vi "R30_1-FPGA.vi"() -> ()   [LabVIEW 2016]
uses:
  Glassman Control.ctl
  Faraday Cup Readback.ctl
  Aperture Readback.ctl
  Gate Valve Readback.ctl
  Glassman Readback.ctl
  <vilib>/LabVIEW Targets/FPGA/cRIO/shared/nicrio_ModuleControls/nicrio_cRIO-9871_BaudRateEnum.ctl
  <vilib>/LabVIEW Targets/FPGA/cRIO/shared/nicrio_ModuleControls/nicrio_cRIO-9871_ParityEnum.ctl
  <vilib>/LabVIEW Targets/FPGA/cRIO/shared/nicrio_ModuleControls/nicrio_cRIO-9871_StopBitsEnum.ctl
  <vilib>/LabVIEW Targets/FPGA/cRIO/shared/nicrio_ModuleControls/nicrio_cRIO-9871_DataBitsEnum.ctl
  <vilib>/Platform/TimedLoop/XDataNode/timing_clust.ctl
  <vilib>/Platform/TimedLoop/XDataNode/nitl_modes.ctl
  <vilib>/Platform/TimedLoop/XDataNode/wakeup.ctl
  <vilib>/rvi/FXPMathLib/basic elements/FxpIntAccumulator/subVIs/nifxpmath_IntAccumulator_SimConfig.ctl
  <vilib>/rvi/Emulation/niFpgaGetClockAttributes.vi
  <vilib>/rvi/Emulation/niFpgaSctlEmulationGetInTimedLoop.vi
  <vilib>/rvi/Emulation/niFpgaEmulationReportErrorSimple.vi
  <vilib>/rvi/eio/common/nirviEmuTemplateMethod_errors.vi
  <vilib>/rvi/Analysis/common/codeGenErrors/XNode/niFpgaXNodeCodeGenErrorHandle.vi
  <vilib>/rvi/Emulation/niFpgaCriticalErrorInLSC.vi
  <vilib>/rvi/FXPMathLib/basic elements/FxpIntAccumulator/simVIs/DllFxpIntAccumulator_sub.vi
  <vilib>/rvi/eio/common/nirviEmuTemplatePropertySet_errors.vi
  <vilib>/eio/EIONode/EIONode.xnode
  <vilib>/rvi/Analysis/measure/dc-rms/XNode/niFpgaDC-RMS.xnode
  <vilib>/Platform/TimedLoop/XDataNode/XDataNode.xnode
  <vilib>/rvi/FXPMathLib/basic elements/FxpIntAccumulator/XNode/nifxpmath_IntAccumulator.xnode
  <vilib>/rvi/FXPMathLib/FxpMul/XNode/nifxpmath_Multiplier.xnode
  <vilib>/eio/EIOPropertyNode/EIOPropertyNode.xnode
  <vilib>/eio/EIOMethodNode/EIOMethodNode.xnode
  <vilib>/Platform/TimedLoop/XDataNode/XDNodeRunTimeDep.lvlib
  <vilib>/rvi/FXPMathLib/sim/FxpSim.dll
  <vilib>/rvi/eio/common/nirviEmuTemplatePropertyGet_errors.vi
  <vilib>/rvi/eio/common/nirviEmuTemplatePropertyGet_noerrors.vi
  <vilib>/rvi/eio/common/nirviEmuTemplatePropertySet_noerrors.vi
panel:
  out "HV readback loop error":errorcluster
  out "Quad B I read":fxp<+/-,26,5>
  out "Quad A I read":fxp<+/-,26,5>
  out "ESA- Monitor":T1
  out "Mag Steerer Monitor":T1
  out "Y- Steerer Monitor":T1
  out "ESA+ Monitor":T1
  out "X+ Steerer Monitor":T1
  out "X- Steerer Monitor":T1
  out "Y+ Steerer Monitor":T1
  in  "RT error":bool
  out "GV Interlock loop error":errorcluster
  out "Vac cluster 3 Interlock":bool
  out "Vac cluster 2 Interlock":bool
  out "Vac cluster 1 Interlock":bool
  in  "Turbo 2 GV Actuator":bool
  in  "Beamline GV 2 Actuator":bool
  in  "Cryo Pump GV Actuator":bool
  in  "Beamline GV 1 Actuator":bool
  in  "Turbo 1 GV Actuator":bool
  in  "Switch Magnet GV Actuator":bool
  out "GV Status Loop error":errorcluster
  out "Cryo Pump GV Status":T2
  out "Turbo 2 GV Status":T2
  out "Beamline GV 2 Status":T2
  out "Turbo 1 GV Status":T2
  out "Beamline GV 1 Status":T2
  out "Switching Mag GV Status":T2
  in  "ESA- HV Enable":bool
  in  "ESA+ HV Enable":bool
  out "Switch Magnet Aperture Position":T3
  out "Detector Aperture Position":T3
  out "Detector FC Position":T4
  out "Switch Magnet FC Position":T4
  out "Actuator loop error":errorcluster
  in  "Y- Steerer V set":T5
  in  "Y+ Steerer V set":T5
  in  "X- Steerer V set":T5
  in  "X+ Steerer V set":T5
  in  "Quad B set":fxp<+/-,20,5>
  in  "Quad A set":fxp<+/-,20,5>
  in  "ESA Voltage set":fxp<+/-,20,5>
  out "HV control loop error":errorcluster
  out "Cryo Readback error":errorcluster
  out "Vacuum Gauge 1 error":errorcluster
  out "Vacuum Gauge 2 error":errorcluster
  out "Vacuum Gauge 3 error":errorcluster
  out "Switch Image Ion Gauge 1":u8[](array[numeric])
  out "Switch Image Convectron 1":u8[](array[numeric])
  out "Time since repurge":u8[](array[numeric])
  out "1st stage temp(k)":u8[](array[numeric])
  out "2nd stage":u8[](array[numeric])
  out "Time since pump on":u8[](array[numeric])
  out "Pump On":u8[](array[numeric])
  out "R30 ESA Convectron  1":u8[](array[numeric])
  out "R30 ESA Ion gauge 1":u8[](array[numeric])
  out "R30 Detector Convectron  1":u8[](array[numeric])
  out "R30 Detector Ion gauge 1":u8[](array[numeric])
  in  "Mag Steerer I-program":fxp<+/-,20,5> format="%.17g"
  in  "Switch magnet Aperture Actuator":bool
  in  "Detector Aperture Actuator":bool
  in  "Detector FC Actuator":bool
  in  "Switch magnet FC Actuator":bool
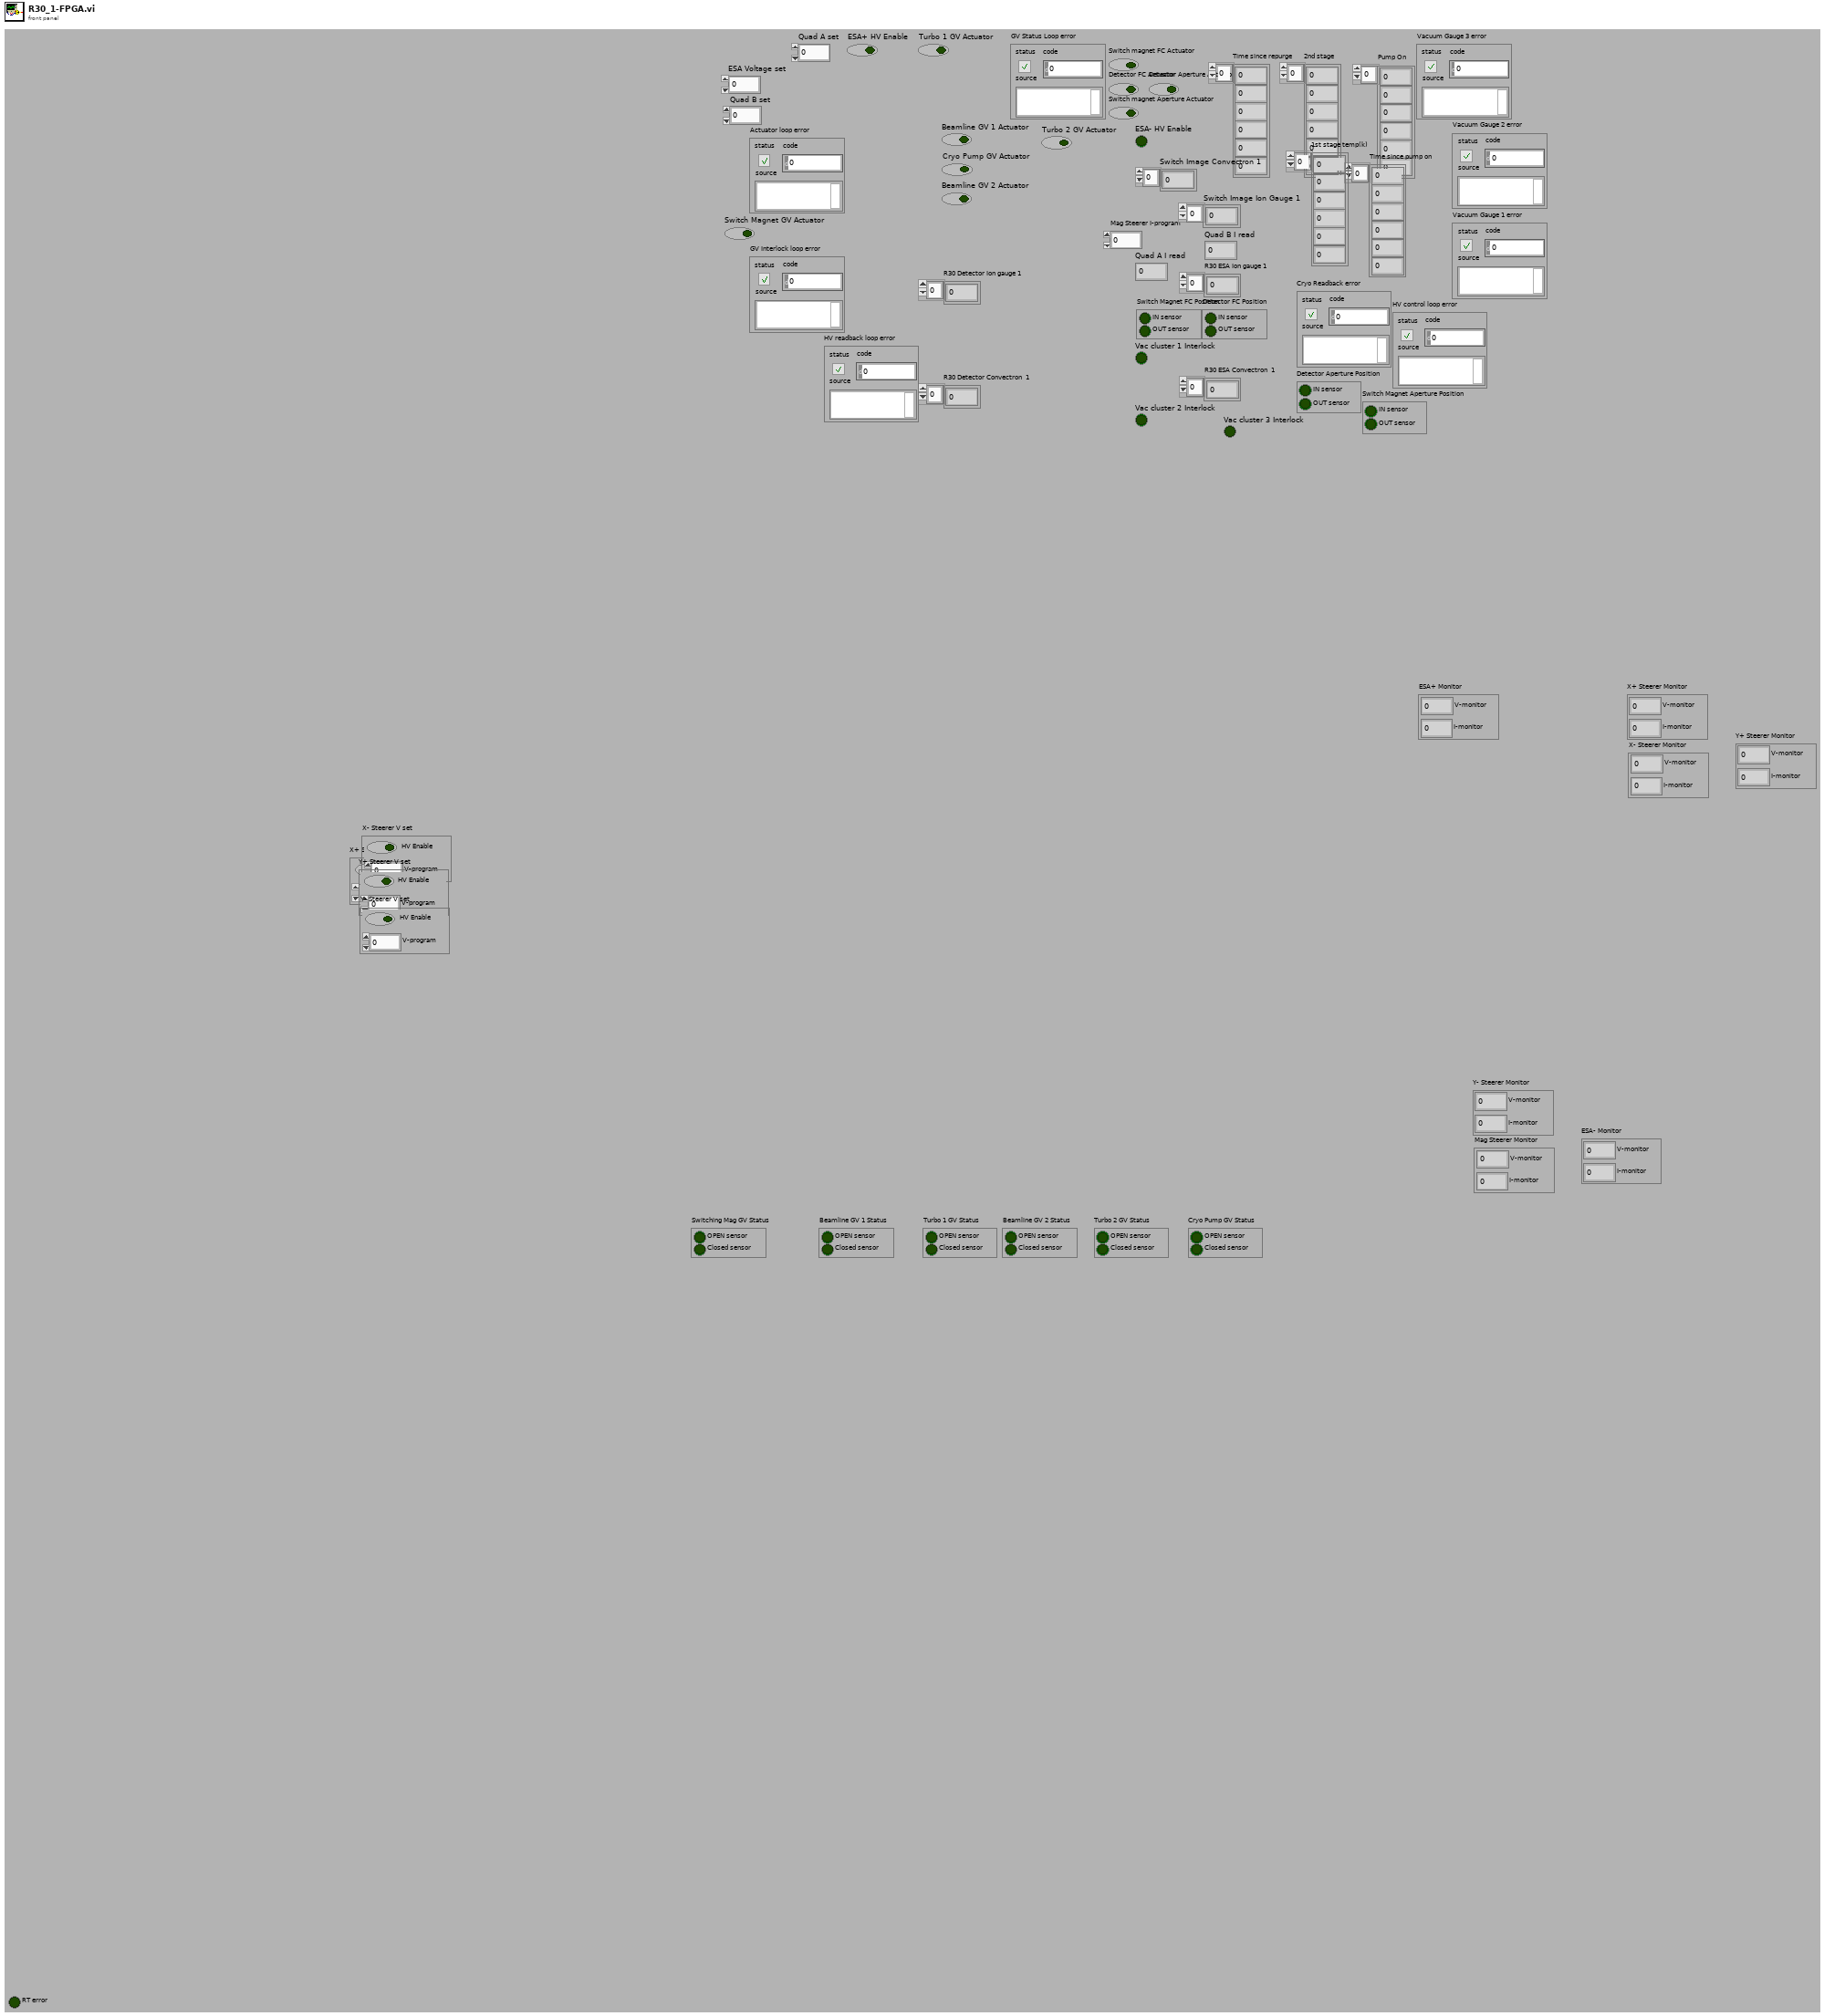
[diagram p1: front panel]
types:
  T1 = typedef "Glassman Readback.ctl" = cluster{"I-monitor":fxp<+/-,26,5>, "V-monitor":fxp<+/-,26,7>}
  T2 = typedef "Gate Valve Readback.ctl" = cluster{"OPEN sensor":bool, "Closed sensor":bool}
  T3 = typedef "Aperture Readback.ctl" = cluster{"IN sensor":bool, "OUT sensor":bool}
  T4 = typedef "Faraday Cup Readback.ctl" = cluster{"IN sensor":bool, "OUT sensor":bool}
  T5 = typedef "Glassman Control.ctl" = cluster{"V-program":fxp<+/-,20,7>, "HV Enable":bool}
  T6 = typedef "nicrio_cRIO-9871_StopBitsEnum.ctl" = enum8{"1", "1.5", "2"}
  T7 = typedef "nicrio_cRIO-9871_ParityEnum.ctl" = enum8{"None", "Odd", "Even", "Mark", "Space"}
  T8 = typedef "nicrio_cRIO-9871_DataBitsEnum.ctl" = enum8{"5", "6", "7", "8"}
  T9 = typedef "nicrio_cRIO-9871_BaudRateEnum.ctl" = enum16{"75 bps", "110 bps", "134 bps", "150 bps", "300 bps", "600 bps", "1200 bps", "1800 bps", "2400 bps", "4800 bps", "7200 bps", "9600 bps", "14.4 kbps", "19.2 kbps", "28.8 kbps", "38.4 kbps", "57.6 kbps", "115.2 kbps", "230.4 kbps", "460.8 kbps", "921.6 kbps"}
  T10 = typedef "XDNodeRunTimeDep.lvlib/timing_clust.ctl" = cluster{"Expected End [f-1]":u64, "Actual End [f-1]":u64, "Finished Late? [f-1]":bool, "Expected End [i-1]":u64, "Actual End [i-1]":u64, "Finished Late? [i-1]":bool, "Expected Start [i]":u64, "Actual Start [i]":u64, "Expected Start [f]":u64, "Actual Start [f]":u64, "Source Name":string, "Structure Name":string, "Period":i64, "Deadline":i64, "Offset":i64, "Start":i64, "Priority":i32, "Timeout":i32, "Mode":T11, "Wakeup Reason":T12, "Error":errorcluster, "Source Type":string, "Secondary Source Type":string, "Global End Time":u64, "Global Start Time":u64, "Frame Duration":u64, "Iteration Duration":u64, "Assigned CPU":i32, "I/O Scan Engine Mode":u32}
  T11 = typedef "XDNodeRunTimeDep.lvlib/nitl_modes.ctl" = enum32{"No Change", "Process missed periods, maintain original phase", "Discard missed periods, maintain original phase", "Process missed periods, ignore original phase", "Discard missed periods, ignore original phase"}
  T12 = typedef "XDNodeRunTimeDep.lvlib/wakeup.ctl" = enum32{"Normal", "Aborted", "Asynchronous wakeup", "Timing source error", "Timed loop error", "Timeout"}
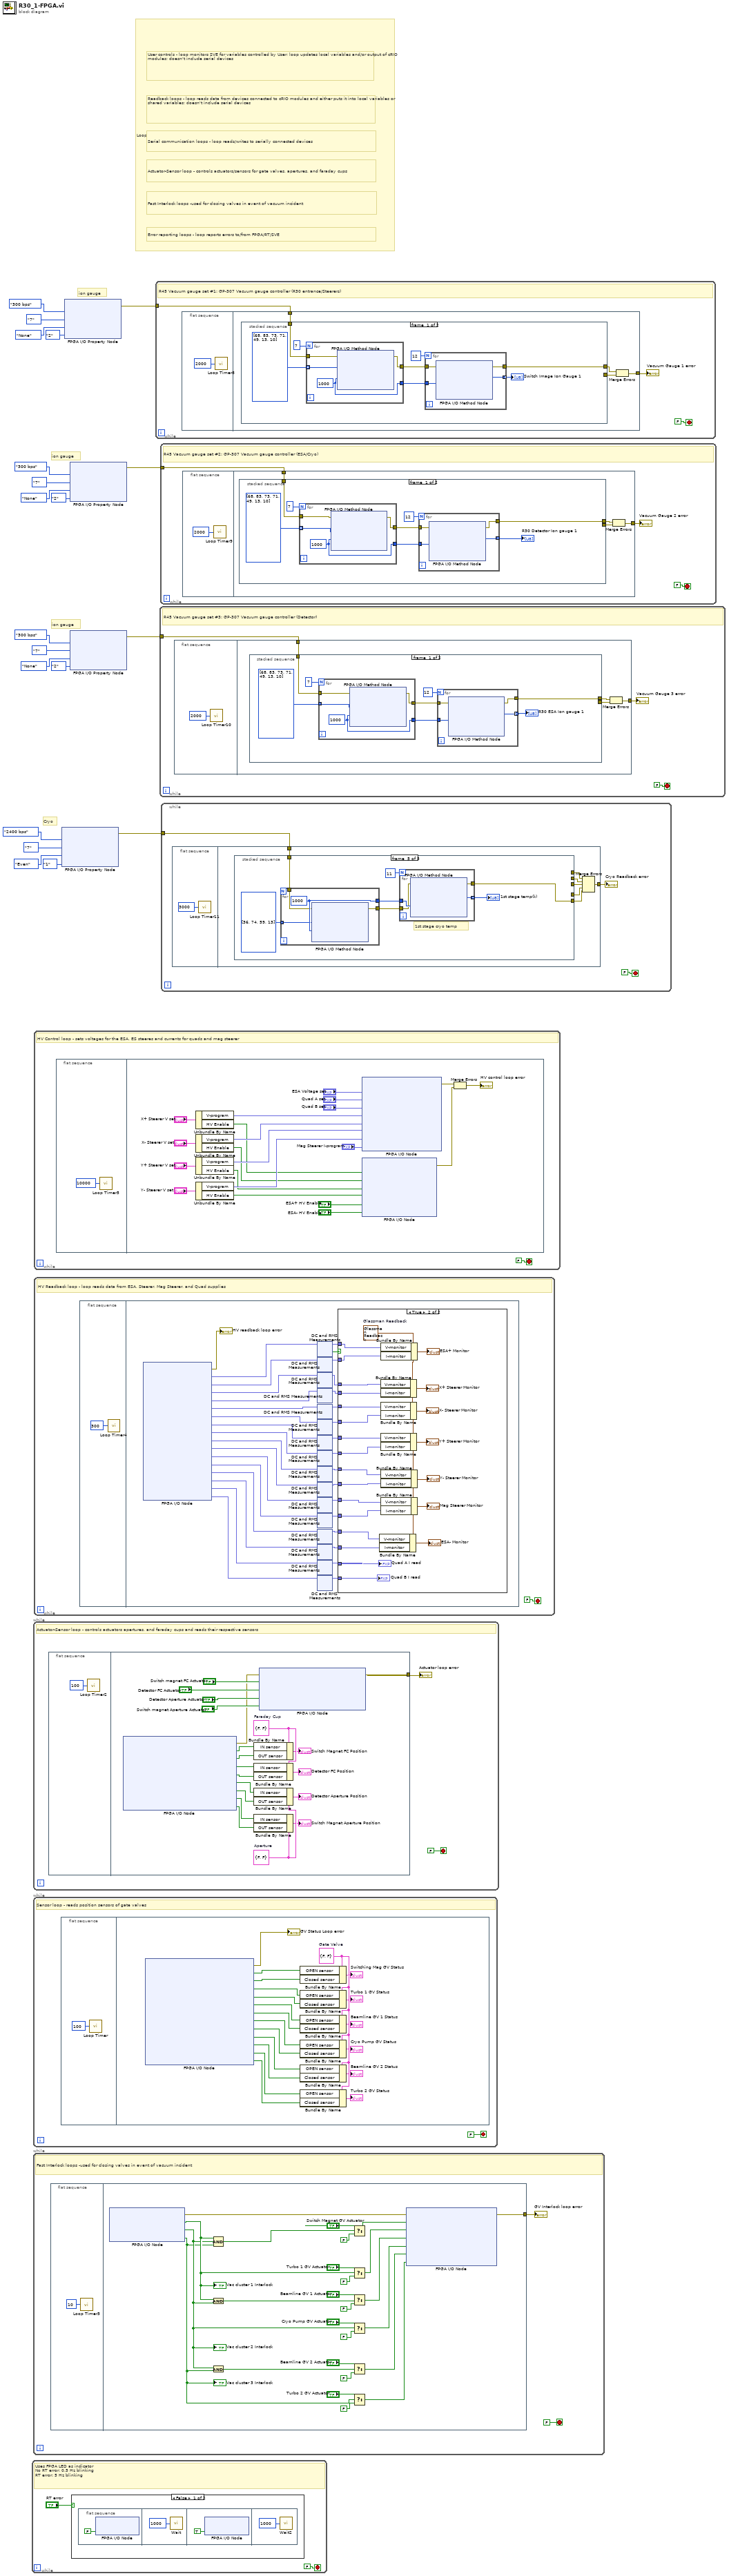
[diagram p0: block diagram]
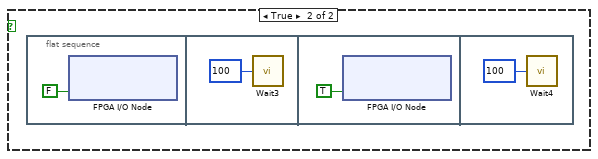
[diagram p2: hidden frame]
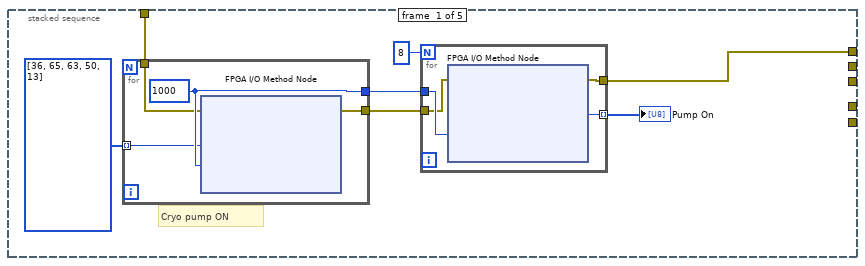
[diagram p3: hidden frame]
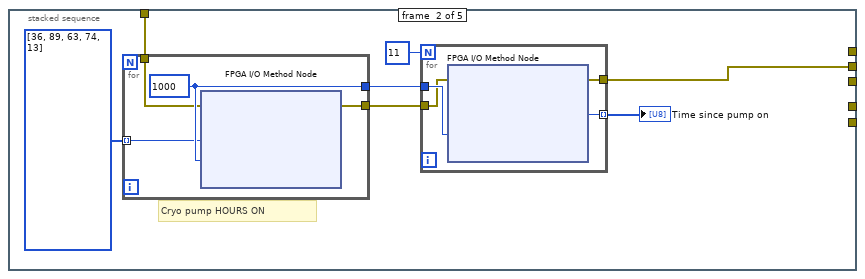
[diagram p4: hidden frame]
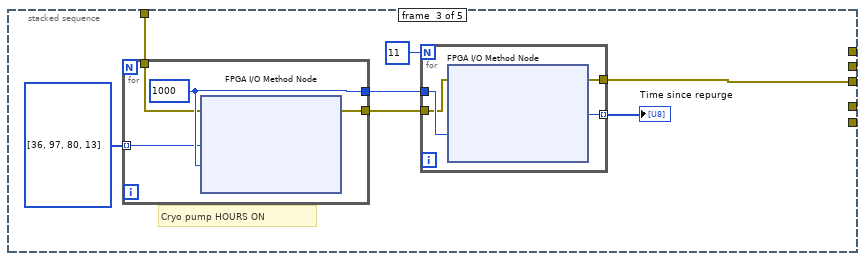
[diagram p5: hidden frame]
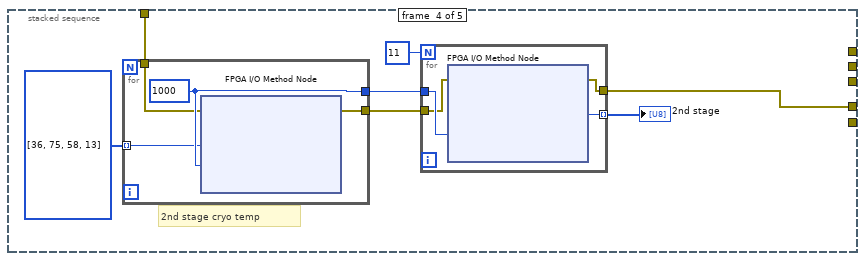
[diagram p6: hidden frame]
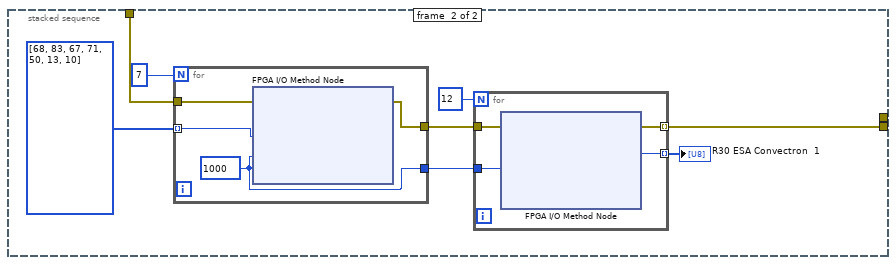
[diagram p7: hidden frame]
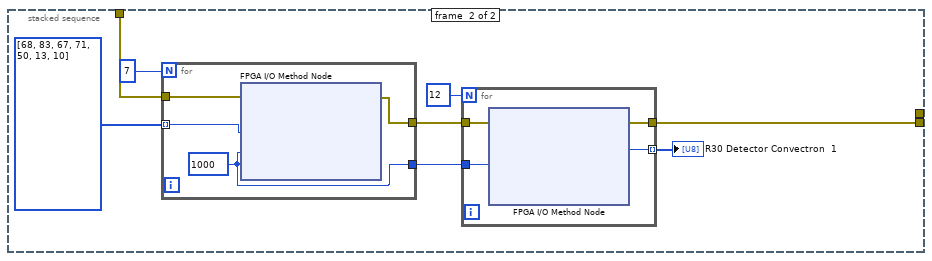
[diagram p8: hidden frame]
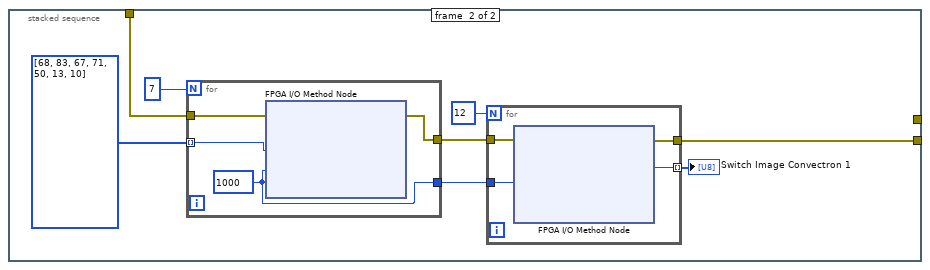
[diagram p9: hidden frame]
diagram:
  # "Actuator-Sensor loop - controls actuators/sensors for gate valves, apertures, and faraday cups"
  # "Fast Interlock loops -used for closing valves in event of vacuum incident"
  # "Error reporting loops - loop reports errors to/from FPGA/RT/SVE"
  # "Serial communication loops - loop reads/writes to serially connected devices"
  # "Readback loops - loop reads data from devices connected to cRIO modules and either puts it into local variables or shared variables; doesn't include serial devices"
  # "User controls - loop monitors SVE for variables controlled by User; loop updates local variables and/or output of cRIO modules; doesn't include serial devices"
  # "Loop legend - loops are color coded by responsibility"
  # "Cryo"
  # "ion gauge"
  # "ion gauge"
  # "ion gauge"
  n1 = while {
    stop <- FALSE stop-if-true
    # "Uses FPGA LED as indicator\nNo RT error: 0.5 Hz blinking\nRT error: 5 Hz blinking"
    n2 = case shown="False" "RT error" {
      frame False {
        n3 = flat-sequence {
          frame #0 {
            n4 = xnode "FPGA I/O Node"("FPGA LED"=FALSE) -> ()  [unwired: 1 in, 1 out]
          }
          frame #1 {
            n5 = call "Wait"("Count(mSec)"=u16 1000) -> ()  [unwired: 1 out]
          }
          frame #2 {
            n6 = xnode "FPGA I/O Node"("FPGA LED"=TRUE) -> ()  [unwired: 1 in, 1 out]
          }
          frame #3 {
            n7 = call "Wait2"("Count(mSec)"=u16 1000) -> ()  [unwired: 1 out]
          }
        }
      }
      frame True {
        n8 = flat-sequence {
          frame #0 {
            n9 = xnode "FPGA I/O Node"("FPGA LED"=FALSE) -> ()  [unwired: 1 in, 1 out]
          }
          frame #1 {
            n10 = call "Wait3"("Count(mSec)"=u16 100) -> ()  [unwired: 1 out]
          }
          frame #2 {
            n11 = xnode "FPGA I/O Node"("FPGA LED"=TRUE) -> ()  [unwired: 1 in, 1 out]
          }
          frame #3 {
            n12 = call "Wait4"("Count(mSec)"=u16 100) -> ()  [unwired: 1 out]
          }
        }
      }
    }
  }
  n13 = while {
    stop <- FALSE stop-if-true
    # "Fast Interlock loops -used for closing valves in event of vacuum incident"
    n14 = flat-sequence {
      tunnel: [w34] -> w31
      frame #0 {
        n15 = call "Loop Timer3"("Count(uSec)"=u32 10) -> ()  [unwired: 1 out]
      }
      frame #1 {
        n16 = xnode "FPGA I/O Node"() -> ("error out"=w59:errorcluster, "Vac cluster 1 Interlock"=w41:bool, "Vac cluster 2 Interlock"=w40:bool, "Vac cluster 3 Interlock"=w39:bool)  [unwired: 4 in, 3 out]
        "Vac cluster 1 Interlock" <- w41
        "Vac cluster 2 Interlock" <- w40
        "Vac cluster 3 Interlock" <- w39
        n17 = And(x=w41, y=w40) -> (x .and. y?=w45:bool)
        n18 = And(x=w40, y=w39) -> (x .and. y?=w52:bool)
        n19 = Compound Arithmetic op=AND(w41, w40, w39) -> (w36:bool)
        n20 = Select(t="Switch Magnet GV Actuator", s=w36, f=FALSE) -> (s? t:f=w35:bool)
        n21 = Select(t="Turbo 1 GV Actuator", s=w41, f=FALSE) -> (s? t:f=w43:bool)
        n22 = Select(t="Beamline GV 1 Actuator", s=w45, f=FALSE) -> (s? t:f=w47:bool)
        n23 = Select(t="Cryo Pump GV Actuator", s=w40, f=FALSE) -> (s? t:f=w50:bool)
        n24 = Select(t="Beamline GV 2 Actuator", s=w52, f=FALSE) -> (s? t:f=w54:bool)
        n25 = Select(t="Turbo 2 GV Actuator", s=w39, f=FALSE) -> (s? t:f=w57:bool)
        n26 = xnode "FPGA I/O Node"("error in"=w59, "Switch Magnet GV Actuator"=w35, "Turbo 1 GV Actuator"=w43, "Beamline GV 1 Actuator"=w47, "Cryo Pump GV Actuator"=w50, "Beamline GV 2 Actuator"=w54, "Turbo 2 GV Actuator"=w57) -> ("error out"=w34:errorcluster)  [unwired: 6 in, 6 out]
      }
    }
    "GV Interlock loop error" <- w31
  }
  n27 = while {
    stop <- FALSE stop-if-true
    # "Actuator-Sensor loop - controls actuators apertures, and faraday cups and reads their respective sensors"
    n28 = flat-sequence {
      tunnel: [w80] -> w60
      frame #0 {
        n29 = call "Loop Timer2"("Count(mSec)"=u32 100 ("Count(uSec)")) -> ()  [unwired: 1 out]
      }
      frame #1 {
        w69 = T3 {"IN sensor"=FALSE, "OUT sensor"=FALSE}  # Aperture
        w72 = T4 {"IN sensor"=FALSE, "OUT sensor"=FALSE}  # Faraday Cup
        n30 = xnode "FPGA I/O Node"() -> ("error out"=w77:errorcluster, "Switch Magnet FC IN sensor"=w76:bool, "Switch Magnet FC OUT sensor"=w75:bool, "Detector FC IN sensor"=w74:bool, "Detector FC OUT sensor"=w73:bool, "Detector Aperture IN sensor"=w65:bool, "Detector Aperture OUT sensor"=w66:bool, "Switch Magnet Aperture IN sensor"=w67:bool, "Switch Magnet Aperture OUT sensor"=w68:bool)  [unwired: 9 in, 8 out]
        n31 = Bundle By Name(cluster=w72, "IN sensor"=w76, "OUT sensor"=w75) -> (→"Switch Magnet FC Position":T4)
        n32 = Bundle By Name(cluster=w72, "IN sensor"=w74, "OUT sensor"=w73) -> (→"Detector FC Position":T4)
        n33 = Bundle By Name(cluster=w69, "IN sensor"=w65, "OUT sensor"=w66) -> (→"Detector Aperture Position":T3)
        n34 = Bundle By Name(cluster=w69, "IN sensor"=w67, "OUT sensor"=w68) -> (→"Switch Magnet Aperture Position":T3)
        n35 = xnode "FPGA I/O Node"("error in"=w77, "Switch Magnet FC Actuator"="Switch magnet FC Actuator", "Detector FC Actuator"="Detector FC Actuator", "Detector Aperture Acutator"="Detector Aperture Actuator", "Switch Magnet Aperture Actuator"="Switch magnet Aperture Actuator") -> ("error out"=w80:errorcluster)  [unwired: 4 in, 4 out]
      }
    }
    "Actuator loop error" <- w60
  }
  n36 = while {
    stop <- FALSE stop-if-true
    # "Sensor loop - reads position sensors of gate valves"
    n37 = flat-sequence {
      frame #0 {
        n38 = call "Loop Timer"("Count(mSec)"=u32 100 ("Count(uSec)")) -> ()  [unwired: 1 out]
      }
      frame #1 {
        w103 = T2 {"OPEN sensor"=FALSE, "Closed sensor"=FALSE}  # Gate Valve
        n39 = xnode "FPGA I/O Node"() -> ("error out"=→"GV Status Loop error":errorcluster, "Swtich Magnet GV OPEN Sensor"=w102:bool, "Swtich Magnet GV CLOSED Sensor"=w101:bool, "Turbo 1 GV OPEN sensor"=w100:bool, "Turbo 1 GV CLOSED sensor"=w99:bool, "Beamline GV 1 OPEN sensor"=w98:bool, "Beamline GV 1 CLOSED sensor"=w97:bool, "Cryo Pump GV OPEN sensor"=w96:bool, "Cryo Pump GV CLOSED sensor"=w95:bool, "Beamline GV 2 OPEN sensor"=w94:bool, "Beamline GV 2 CLOSED sensor"=w93:bool, "Turbo 2 GV OPEN sensor"=w92:bool, "Turbo 2 GV CLOSED sensor"=w91:bool)  [unwired: 13 in, 12 out]
        n40 = Bundle By Name(cluster=w103, "OPEN sensor"=w102, "Closed sensor"=w101) -> (→"Switching Mag GV Status":T2)
        n41 = Bundle By Name(cluster=w103, "OPEN sensor"=w100, "Closed sensor"=w99) -> (→"Turbo 1 GV Status":T2)
        n42 = Bundle By Name(cluster=w103, "OPEN sensor"=w98, "Closed sensor"=w97) -> (→"Beamline GV 1 Status":T2)
        n43 = Bundle By Name(cluster=w103, "OPEN sensor"=w96, "Closed sensor"=w95) -> (→"Cryo Pump GV Status":T2)
        n44 = Bundle By Name(cluster=w103, "OPEN sensor"=w94, "Closed sensor"=w93) -> (→"Beamline GV 2 Status":T2)
        n45 = Bundle By Name(cluster=w103, "OPEN sensor"=w92, "Closed sensor"=w91) -> (→"Turbo 2 GV Status":T2)
      }
    }
  }
  n46 = while {
    stop <- FALSE stop-if-true
    # "HV Control loop - sets voltages for the ESA, ES steeres and currents for quads and mag steerer"
    n47 = flat-sequence {
      frame #0 {
        n48 = call "Loop Timer5"("Count(Ticks)"=u32 10000 ("Count(mSec)")) -> ()  [unwired: 1 out]
      }
      frame #1 {
        n49 = Unbundle By Name("X+ Steerer V set") -> ("V-program"=w118:fxp<+/-,20,7>, "HV Enable"=w111:bool)
        n50 = Unbundle By Name("X- Steerer V set") -> ("V-program"=w117:fxp<+/-,20,7>, "HV Enable"=w112:bool)
        n51 = Unbundle By Name("Y+ Steerer V set") -> ("V-program"=w116:fxp<+/-,20,7>, "HV Enable"=w113:bool)
        n52 = Unbundle By Name("Y- Steerer V set") -> ("V-program"=w115:fxp<+/-,20,7>, "HV Enable"=w114:bool)
        n53 = xnode "FPGA I/O Node"("X+ Steerer HV Enable"=w111, "X- Steerer HV Enable"=w112, "Y+ Steerer HV Enable"=w113, "Y- Steerer HV Enable"=w114, "ESA+ HV Enable"="ESA+ HV Enable", "ESA- HV Enable"="ESA- HV Enable") -> ("error out"=w109:errorcluster)  [unwired: 7 in, 6 out]
        n54 = xnode "FPGA I/O Node"("ESA Voltage set"="ESA Voltage set", "Quad A set"="Quad A set", "Quad B set"="Quad B set", "X+ Steerer V set"=w118, "X- Steerer V set"=w117, "Y+ Steerer V set"=w116, "Y- Steerer V set"=w115, "Mag Steerer I-program"="Mag Steerer I-program") -> ("error out"=w126:errorcluster)  [unwired: 9 in, 8 out]
        n55 = Merge Errors(w126, w109) -> (→"HV control loop error":errorcluster)
      }
    }
  }
  n56 = while {
    stop <- FALSE stop-if-true
    # "HV Readback loop - loop reads data from ESA, Steerer, Mag Steerer, and Quad supplies"
    n57 = flat-sequence {
      frame #0 {
        n58 = call "Loop Timer4"("Count(Ticks)"=u32 300) -> ()  [unwired: 1 out]
      }
      frame #1 {
        n59 = xnode "FPGA I/O Node"() -> ("error out"=→"HV readback loop error":errorcluster, "ESA+ V read"=w154:fxp<+/-,26,5>, "ESA+ I read"=w153:fxp<+/-,26,5>, "X+ Steerer V read"=w152:fxp<+/-,26,5>, "X+ Steerer I read"=w151:fxp<+/-,26,5>, "X- Steerer V read"=w150:fxp<+/-,26,5>, "X- Steerer I read"=w149:fxp<+/-,26,5>, "Y+ Steerer V read"=w148:fxp<+/-,26,5>, "Y+ Steerer I read"=w147:fxp<+/-,26,5>, "Y- Steerer V read"=w140:fxp<+/-,26,5>, "Y- Steerer I read"=w139:fxp<+/-,26,5>, "Mag Steerer V read"=w138:fxp<+/-,26,5>, "Mag Steerer I read"=w137:fxp<+/-,26,5>, "ESA- V read"=w136:fxp<+/-,26,5>, "ESA- I read"=w135:fxp<+/-,26,5>, "Quad A I read"=w134:fxp<+/-,26,5>, "Quad B I read"=w133:fxp<+/-,26,5>)  [unwired: 17 in, 16 out]
        n60 = xnode "DC and RMS Measurements"("input data"=w154) -> ("DC"=w162:fxp<+/-,26,5>, "output valid"=w163:bool)  [unwired: 1 in]
        n61 = xnode "DC and RMS Measurements"("input data"=w153) -> ("DC"=w161:fxp<+/-,26,5>)  [unwired: 1 in, 1 out]
        n62 = xnode "DC and RMS Measurements"("input data"=w152) -> ("DC"=w160:fxp<+/-,26,5>)  [unwired: 1 in, 1 out]
        n63 = xnode "DC and RMS Measurements"("input data"=w151) -> ("DC"=w159:fxp<+/-,26,5>)  [unwired: 1 in, 1 out]
        n64 = xnode "DC and RMS Measurements"("input data"=w150) -> ("DC"=w158:fxp<+/-,26,5>)  [unwired: 1 in, 1 out]
        n65 = xnode "DC and RMS Measurements"("input data"=w149) -> ("DC"=w157:fxp<+/-,26,5>)  [unwired: 1 in, 1 out]
        n66 = xnode "DC and RMS Measurements"("input data"=w148) -> ("DC"=w156:fxp<+/-,26,5>)  [unwired: 1 in, 1 out]
        n67 = xnode "DC and RMS Measurements"("input data"=w147) -> ("DC"=w155:fxp<+/-,26,5>)  [unwired: 1 in, 1 out]
        n68 = xnode "DC and RMS Measurements"("input data"=w140) -> ("DC"=w146:fxp<+/-,26,5>)  [unwired: 1 in, 1 out]
        n69 = xnode "DC and RMS Measurements"("input data"=w139) -> ("DC"=w145:fxp<+/-,26,5>)  [unwired: 1 in, 1 out]
        n70 = xnode "DC and RMS Measurements"("input data"=w138) -> ("DC"=w144:fxp<+/-,26,5>)  [unwired: 1 in, 1 out]
        n71 = xnode "DC and RMS Measurements"("input data"=w137) -> ("DC"=w143:fxp<+/-,26,5>)  [unwired: 1 in, 1 out]
        n72 = xnode "DC and RMS Measurements"("input data"=w136) -> ("DC"=w142:fxp<+/-,26,5>)  [unwired: 1 in, 1 out]
        n73 = xnode "DC and RMS Measurements"("input data"=w135) -> ("DC"=w141:fxp<+/-,26,5>)  [unwired: 1 in, 1 out]
        n74 = xnode "DC and RMS Measurements"("input data"=w134) -> ("DC"=w132:fxp<+/-,26,5>)  [unwired: 1 in, 1 out]
        n75 = xnode "DC and RMS Measurements"("input data"=w133) -> ("DC"=w131:fxp<+/-,26,5>)  [unwired: 1 in, 1 out]
        n76 = case shown="True" w163 {
          tunnel: w162 -> [_ w987]
          tunnel: w161 -> [_ w986]
          tunnel: w160 -> [_ w982]
          tunnel: w159 -> [_ w981]
          tunnel: w158 -> [_ w980]
          tunnel: w157 -> [_ w979]
          tunnel: w156 -> [_ w977]
          tunnel: w155 -> [_ w976]
          tunnel: w146 -> [_ w972]
          tunnel: w145 -> [_ w971]
          tunnel: w144 -> [_ w970]
          tunnel: w143 -> [_ w969]
          tunnel: w142 -> [_ w968]
          tunnel: w141 -> [_ w967]
          tunnel: w132 -> [_ w965]
          tunnel: w131 -> [_ w964]
          frame False {
          }
          frame True {
            w966 = T1 {"I-monitor"=0.0, "V-monitor"=0.0}  # Glassman Readback
            n77 = Bundle By Name(cluster=w966, "V-monitor"=w968, "I-monitor"=w967) -> (→"ESA- Monitor":T1)
            n78 = Bundle By Name(cluster=w966, "V-monitor"=w982, "I-monitor"=w981) -> (→"X+ Steerer Monitor":T1)
            n79 = Bundle By Name(cluster=w966, "V-monitor"=w980, "I-monitor"=w979) -> (→"X- Steerer Monitor":T1)
            n80 = Bundle By Name(cluster=w966, "V-monitor"=w977, "I-monitor"=w976) -> (→"Y+ Steerer Monitor":T1)
            n81 = Bundle By Name(cluster=w966, "V-monitor"=w987, "I-monitor"=w986) -> (→"ESA+ Monitor":T1)
            n82 = Bundle By Name(cluster=w966, "V-monitor"=w972, "I-monitor"=w971) -> (→"Y- Steerer Monitor":T1)
            n83 = Bundle By Name(cluster=w966, "V-monitor"=w970, "I-monitor"=w969) -> (→"Mag Steerer Monitor":T1)
            "Quad A I read" <- w965
            "Quad B I read" <- w964
          }
        }
      }
    }
  }
  n84 = xnode "FPGA I/O Property Node"("Baud Rate"=nicrio_cRIO-9871_BaudRateEnum."2400 bps", "Data Bits"=nicrio_cRIO-9871_DataBitsEnum."7", "Parity"=nicrio_cRIO-9871_ParityEnum."Even", "Stop Bits"=nicrio_cRIO-9871_StopBitsEnum."1") -> ("error out"=w1:errorcluster)  [unwired: 2 in, 1 out]
  n85 = xnode "FPGA I/O Property Node"("Baud Rate"=nicrio_cRIO-9871_BaudRateEnum."300 bps", "Data Bits"=nicrio_cRIO-9871_DataBitsEnum."7", "Parity"=nicrio_cRIO-9871_ParityEnum."None", "Stop Bits"=nicrio_cRIO-9871_StopBitsEnum."2") -> ("error out"=w4:errorcluster)  [unwired: 2 in, 1 out]
  n86 = xnode "FPGA I/O Property Node"("Baud Rate"=nicrio_cRIO-9871_BaudRateEnum."300 bps", "Data Bits"=nicrio_cRIO-9871_DataBitsEnum."7", "Parity"=nicrio_cRIO-9871_ParityEnum."None", "Stop Bits"=nicrio_cRIO-9871_StopBitsEnum."2") -> ("error out"=w3:errorcluster)  [unwired: 2 in, 1 out]
  n87 = xnode "FPGA I/O Property Node"("Baud Rate"=nicrio_cRIO-9871_BaudRateEnum."300 bps", "Data Bits"=nicrio_cRIO-9871_DataBitsEnum."7", "Parity"=nicrio_cRIO-9871_ParityEnum."None", "Stop Bits"=nicrio_cRIO-9871_StopBitsEnum."2") -> ("error out"=w2:errorcluster)  [unwired: 2 in, 1 out]
  n88 = while {
    tunnel: w4 -> [w1469]
    stop <- FALSE stop-if-true
    # "R45 Vacuum gauge set #1: GP-307 Vacuum gauge controller (R30 entrance/Steerers)"
    n89 = flat-sequence {
      tunnel: w1469 -> [w1475]
      tunnel: [w1472] -> w1468
      frame #0 {
        n90 = call "Loop Timer8"("Count(mSec)"=u32 2000 ("Count(Ticks)")) -> ()  [unwired: 1 out]
      }
      frame #1 {
        n91 = stacked-sequence {
          tunnel: w1475 -> [w1478 w1494]
          tunnel: [_ w1492] -> w1474
          tunnel: [w1476 _] -> w1473
          frame #0 {
            n92 = for {
              N: 7 -> [_]
              tunnel: [w1490] -> w1483
              tunnel: u8[] [68, 83, 73, 71, 49, 13, 10] ("unsigned byte array") -> [w1491] mode=indexing
              tunnel: w1478 -> [w1489]
              tunnel: [w1488] -> w1477
              w1490 = 1000 ("Timeout (ms)")
              n93 = xnode "FPGA I/O Method Node"("error in"=w1489, "Data"=w1491, "Timeout (ms)"=w1490) -> ("error out"=w1488:errorcluster)  [unwired: 1 in, 2 out]
            }
            n94 = for {
              N: 12 -> [_]
              tunnel: w1483 -> [w1487]
              tunnel: [w1486] -> w1479 mode=indexing
              tunnel: w1477 -> [w1485]
              tunnel: [w1484] -> w1476
              n95 = xnode "FPGA I/O Method Node"("error in"=w1485, "Timeout (ms)"=w1487) -> ("error out"=w1484:errorcluster, "Data"=w1486:u8)  [unwired: 1 in, 2 out]
            }
            "Switch Image Ion Gauge 1" <- w1479
          }
          frame #1 {
            n96 = for {
              N: 7 -> [_]
              tunnel: [w1506] -> w1499
              tunnel: u8[] [68, 83, 67, 71, 50, 13, 10] ("unsigned byte array") -> [w1507] mode=indexing
              tunnel: w1494 -> [w1505]
              tunnel: [w1504] -> w1493
              w1506 = 1000 ("Timeout (ms)")
              n97 = xnode "FPGA I/O Method Node"("error in"=w1505, "Data"=w1507, "Timeout (ms)"=w1506) -> ("error out"=w1504:errorcluster)  [unwired: 1 in, 2 out]
            }
            n98 = for {
              N: 12 -> [_]
              tunnel: w1499 -> [w1503]
              tunnel: [w1502] -> w1495 mode=indexing
              tunnel: w1493 -> [w1501]
              tunnel: [w1500] -> w1492
              n99 = xnode "FPGA I/O Method Node"("error in"=w1501, "Timeout (ms)"=w1503) -> ("error out"=w1500:errorcluster, "Data"=w1502:u8)  [unwired: 1 in, 2 out]
            }
            "Switch Image Convectron 1" <- w1495
          }
        }
        n100 = Merge Errors(w1473, w1474) -> (w1472:errorcluster)
      }
    }
    "Vacuum Gauge 1 error" <- w1468
  }
  n101 = while {
    tunnel: w2 -> [w1509]
    stop <- FALSE stop-if-true
    # "R45 Vacuum gauge set #3: GP-307 Vacuum gauge controller (Detector)"
    n102 = flat-sequence {
      tunnel: w1509 -> [w1515]
      tunnel: [w1512] -> w1508
      frame #0 {
        n103 = call "Loop Timer10"("Count(mSec)"=u32 2000 ("Count(Ticks)")) -> ()  [unwired: 1 out]
      }
      frame #1 {
        n104 = stacked-sequence {
          tunnel: w1515 -> [w1518 w1534]
          tunnel: [_ w1532] -> w1514
          tunnel: [w1516 _] -> w1513
          frame #0 {
            n105 = for {
              N: 7 -> [_]
              tunnel: [w1530] -> w1523
              tunnel: u8[] [68, 83, 73, 71, 49, 13, 10] ("unsigned byte array") -> [w1531] mode=indexing
              tunnel: w1518 -> [w1529]
              tunnel: [w1528] -> w1517
              w1530 = 1000 ("Timeout (ms)")
              n106 = xnode "FPGA I/O Method Node"("error in"=w1529, "Data"=w1531, "Timeout (ms)"=w1530) -> ("error out"=w1528:errorcluster)  [unwired: 1 in, 2 out]
            }
            n107 = for {
              N: 12 -> [_]
              tunnel: w1523 -> [w1527]
              tunnel: [w1526] -> w1519 mode=indexing
              tunnel: w1517 -> [w1525]
              tunnel: [w1524] -> w1516
              n108 = xnode "FPGA I/O Method Node"("error in"=w1525, "Timeout (ms)"=w1527) -> ("error out"=w1524:errorcluster, "Data"=w1526:u8)  [unwired: 1 in, 2 out]
            }
            "R30 ESA Ion gauge 1" <- w1519
          }
          frame #1 {
            n109 = for {
              N: 7 -> [_]
              tunnel: [w1546] -> w1539
              tunnel: u8[] [68, 83, 67, 71, 50, 13, 10] ("unsigned byte array") -> [w1547] mode=indexing
              tunnel: w1534 -> [w1545]
              tunnel: [w1544] -> w1533
              w1546 = 1000 ("Timeout (ms)")
              n110 = xnode "FPGA I/O Method Node"("error in"=w1545, "Data"=w1547, "Timeout (ms)"=w1546) -> ("error out"=w1544:errorcluster)  [unwired: 1 in, 2 out]
            }
            n111 = for {
              N: 12 -> [_]
              tunnel: w1539 -> [w1543]
              tunnel: [w1542] -> w1535 mode=indexing
              tunnel: w1533 -> [w1541]
              tunnel: [w1540] -> w1532 mode=indexing
              n112 = xnode "FPGA I/O Method Node"("error in"=w1541, "Timeout (ms)"=w1543) -> ("error out"=w1540:errorcluster, "Data"=w1542:u8)  [unwired: 1 in, 2 out]
            }
            "R30 ESA Convectron  1" <- w1535
          }
        }
        n113 = Merge Errors(w1513, w1514) -> (w1512:errorcluster)
      }
    }
    "Vacuum Gauge 3 error" <- w1508
  }
  n114 = while {
    tunnel: w3 -> [w1549]
    stop <- FALSE stop-if-true
    # "R45 Vacuum gauge set #2: GP-307 Vacuum gauge controller (ESA/Cryo)"
    n115 = flat-sequence {
      tunnel: w1549 -> [w1555]
      tunnel: [w1552] -> w1548
      frame #0 {
        n116 = call "Loop Timer9"("Count(mSec)"=u32 2000 ("Count(Ticks)")) -> ()  [unwired: 1 out]
      }
      frame #1 {
        n117 = stacked-sequence {
          tunnel: w1555 -> [w1558 w1574]
          tunnel: [_ w1572] -> w1554
          tunnel: [w1556 _] -> w1553
          frame #0 {
            n118 = for {
              N: 7 -> [_]
              tunnel: [w1570] -> w1563
              tunnel: u8[] [68, 83, 73, 71, 49, 13, 10] ("unsigned byte array") -> [w1571] mode=indexing
              tunnel: w1558 -> [w1569]
              tunnel: [w1568] -> w1557
              w1570 = 1000 ("Timeout (ms)")
              n119 = xnode "FPGA I/O Method Node"("error in"=w1569, "Data"=w1571, "Timeout (ms)"=w1570) -> ("error out"=w1568:errorcluster)  [unwired: 1 in, 2 out]
            }
            n120 = for {
              N: 12 -> [_]
              tunnel: w1563 -> [w1567]
              tunnel: [w1566] -> w1559 mode=indexing
              tunnel: w1557 -> [w1565]
              tunnel: [w1564] -> w1556
              n121 = xnode "FPGA I/O Method Node"("error in"=w1565, "Timeout (ms)"=w1567) -> ("error out"=w1564:errorcluster, "Data"=w1566:u8)  [unwired: 1 in, 2 out]
            }
            "R30 Detector Ion gauge 1" <- w1559
          }
          frame #1 {
            n122 = for {
              N: 7 -> [_]
              tunnel: [w1586] -> w1579
              tunnel: u8[] [68, 83, 67, 71, 50, 13, 10] ("unsigned byte array") -> [w1587] mode=indexing
              tunnel: w1574 -> [w1585]
              tunnel: [w1584] -> w1573
              w1586 = 1000 ("Timeout (ms)")
              n123 = xnode "FPGA I/O Method Node"("error in"=w1585, "Data"=w1587, "Timeout (ms)"=w1586) -> ("error out"=w1584:errorcluster)  [unwired: 1 in, 2 out]
            }
            n124 = for {
              N: 12 -> [_]
              tunnel: w1579 -> [w1583]
              tunnel: [w1582] -> w1575 mode=indexing
              tunnel: w1573 -> [w1581]
              tunnel: [w1580] -> w1572
              n125 = xnode "FPGA I/O Method Node"("error in"=w1581, "Timeout (ms)"=w1583) -> ("error out"=w1580:errorcluster, "Data"=w1582:u8)  [unwired: 1 in, 2 out]
            }
            "R30 Detector Convectron  1" <- w1575
          }
        }
        n126 = Merge Errors(w1553, w1554) -> (w1552:errorcluster)
      }
    }
    "Vacuum Gauge 2 error" <- w1548
  }
  n127 = while {
    tunnel: w1 -> [w1589]
    stop <- FALSE stop-if-true
    n128 = flat-sequence {
      tunnel: w1589 -> [w1598]
      tunnel: [w1592] -> w1588
      frame #0 {
        n129 = call "Loop Timer11"("Count(mSec)"=u32 3000 ("Count(Ticks)")) -> ()  [unwired: 1 out]
      }
      frame #1 {
        n130 = stacked-sequence {
          tunnel: w1598 -> [w1600 w1615 w1631 w1646 w1661]
          tunnel: [w1601 _ _ _ _] -> w1597
          tunnel: [_ w1616 _ _ _] -> w1596
          tunnel: [_ _ w1629 _ _] -> w1595
          tunnel: [_ _ _ w1644 _] -> w1594
          tunnel: [_ _ _ _ w1659] -> w1593
          frame #0 {
            # "Cryo pump ON"
            n131 = for {
              tunnel: [w1613] -> w1605
              tunnel: u8[] [36, 65, 63, 50, 13] ("unsigned byte array") -> [w1612] mode=indexing
              tunnel: w1600 -> [w1611]
              tunnel: [w1610] -> w1599
              w1613 = 1000 ("Timeout (ms)")
              n132 = xnode "FPGA I/O Method Node"("error in"=w1611, "Data"=w1612, "Timeout (ms)"=w1613) -> ("error out"=w1610:errorcluster)  [unwired: 1 in, 2 out]
            }
            n133 = for {
              N: 8 -> [_]
              tunnel: w1605 -> [w1609]
              tunnel: [w1608] -> w1602 mode=indexing
              tunnel: [w1607] -> w1601
              tunnel: w1599 -> [w1606]
              n134 = xnode "FPGA I/O Method Node"("error in"=w1606, "Timeout (ms)"=w1609) -> ("error out"=w1607:errorcluster, "Data"=w1608:u8)  [unwired: 1 in, 2 out]
            }
            "Pump On" <- w1602
          }
          frame #1 {
            # "Cryo pump HOURS ON"
            n135 = for {
              tunnel: [w1628] -> w1620
              tunnel: u8[] [36, 89, 63, 74, 13] ("unsigned byte array") -> [w1627] mode=indexing
              tunnel: w1615 -> [w1626]
              tunnel: [w1625] -> w1614
              w1628 = 1000 ("Timeout (ms)")
              n136 = xnode "FPGA I/O Method Node"("error in"=w1626, "Data"=w1627, "Timeout (ms)"=w1628) -> ("error out"=w1625:errorcluster)  [unwired: 1 in, 2 out]
            }
            n137 = for {
              N: 11 -> [_]
              tunnel: w1620 -> [w1624]
              tunnel: [w1623] -> w1617 mode=indexing
              tunnel: [w1622] -> w1616
              tunnel: w1614 -> [w1621]
              n138 = xnode "FPGA I/O Method Node"("error in"=w1621, "Timeout (ms)"=w1624) -> ("error out"=w1622:errorcluster, "Data"=w1623:u8)  [unwired: 1 in, 2 out]
            }
            "Time since pump on" <- w1617
          }
          frame #2 {
            # "Cryo pump HOURS ON"
            n139 = for {
              tunnel: [w1643] -> w1635
              tunnel: u8[] [36, 97, 80, 13] ("unsigned byte array") -> [w1642] mode=indexing
              tunnel: w1631 -> [w1641]
              tunnel: [w1640] -> w1630
              w1643 = 1000 ("Timeout (ms)")
              n140 = xnode "FPGA I/O Method Node"("error in"=w1641, "Data"=w1642, "Timeout (ms)"=w1643) -> ("error out"=w1640:errorcluster)  [unwired: 1 in, 2 out]
            }
            n141 = for {
              N: 11 -> [_]
              tunnel: w1635 -> [w1639]
              tunnel: [w1638] -> w1632 mode=indexing
              tunnel: w1630 -> [w1637]
              tunnel: [w1636] -> w1629
              n142 = xnode "FPGA I/O Method Node"("error in"=w1637, "Timeout (ms)"=w1639) -> ("error out"=w1636:errorcluster, "Data"=w1638:u8)  [unwired: 1 in, 2 out]
            }
            "Time since repurge" <- w1632
          }
          frame #3 {
            # "2nd stage cryo temp"
            n143 = for {
              tunnel: [w1658] -> w1650
              tunnel: u8[] [36, 75, 58, 13] ("unsigned byte array") -> [w1657] mode=indexing
              tunnel: w1646 -> [w1656]
              tunnel: [w1655] -> w1645
              w1658 = 1000 ("Timeout (ms)")
              n144 = xnode "FPGA I/O Method Node"("error in"=w1656, "Data"=w1657, "Timeout (ms)"=w1658) -> ("error out"=w1655:errorcluster)  [unwired: 1 in, 2 out]
            }
            n145 = for {
              N: 11 -> [_]
              tunnel: w1650 -> [w1654]
              tunnel: [w1653] -> w1647 mode=indexing
              tunnel: w1645 -> [w1652]
              tunnel: [w1651] -> w1644
              n146 = xnode "FPGA I/O Method Node"("error in"=w1652, "Timeout (ms)"=w1654) -> ("error out"=w1651:errorcluster, "Data"=w1653:u8)  [unwired: 1 in, 2 out]
            }
            "2nd stage" <- w1647
          }
          frame #4 {
            # "1st stage cryo temp"
            n147 = for {
              tunnel: [w1673] -> w1665
              tunnel: u8[] [36, 74, 59, 13] ("unsigned byte array") -> [w1672] mode=indexing
              tunnel: w1661 -> [w1671]
              tunnel: [w1670] -> w1660
              w1673 = 1000 ("Timeout (ms)")
              n148 = xnode "FPGA I/O Method Node"("error in"=w1671, "Data"=w1672, "Timeout (ms)"=w1673) -> ("error out"=w1670:errorcluster)  [unwired: 1 in, 2 out]
            }
            n149 = for {
              N: 11 -> [_]
              tunnel: w1665 -> [w1669]
              tunnel: [w1668] -> w1662 mode=indexing
              tunnel: w1660 -> [w1667]
              tunnel: [w1666] -> w1659
              n150 = xnode "FPGA I/O Method Node"("error in"=w1667, "Timeout (ms)"=w1669) -> ("error out"=w1666:errorcluster, "Data"=w1668:u8)  [unwired: 1 in, 2 out]
            }
            "1st stage temp(k)" <- w1662
          }
        }
        n151 = Merge Errors(w1597, w1596, w1595, w1594, w1593) -> (w1592:errorcluster)
      }
    }
    "Cryo Readback error" <- w1588
  }
